vi "Seq Edit Step.vi"(6 "config paths":T1, 8 "Error In":errorcluster, 9 "Segment Info In":T2, 10 "Basic Steps":string[](array[string]), 11 "VI Names":string[](array[string])) -> (0 "Error Out":errorcluster, 1 "Step Hisitory":string[](array[string]), 2 "Segment Info Out":T2, 3 "Add Step?":bool)   [LabVIEW 2018]
uses:
  type defs/Sequence Info.ctl
  type defs/config paths for seq def.ctl
panel:
  out "File Name":string
  out "file or folder exists?":bool
  out "appended path":path
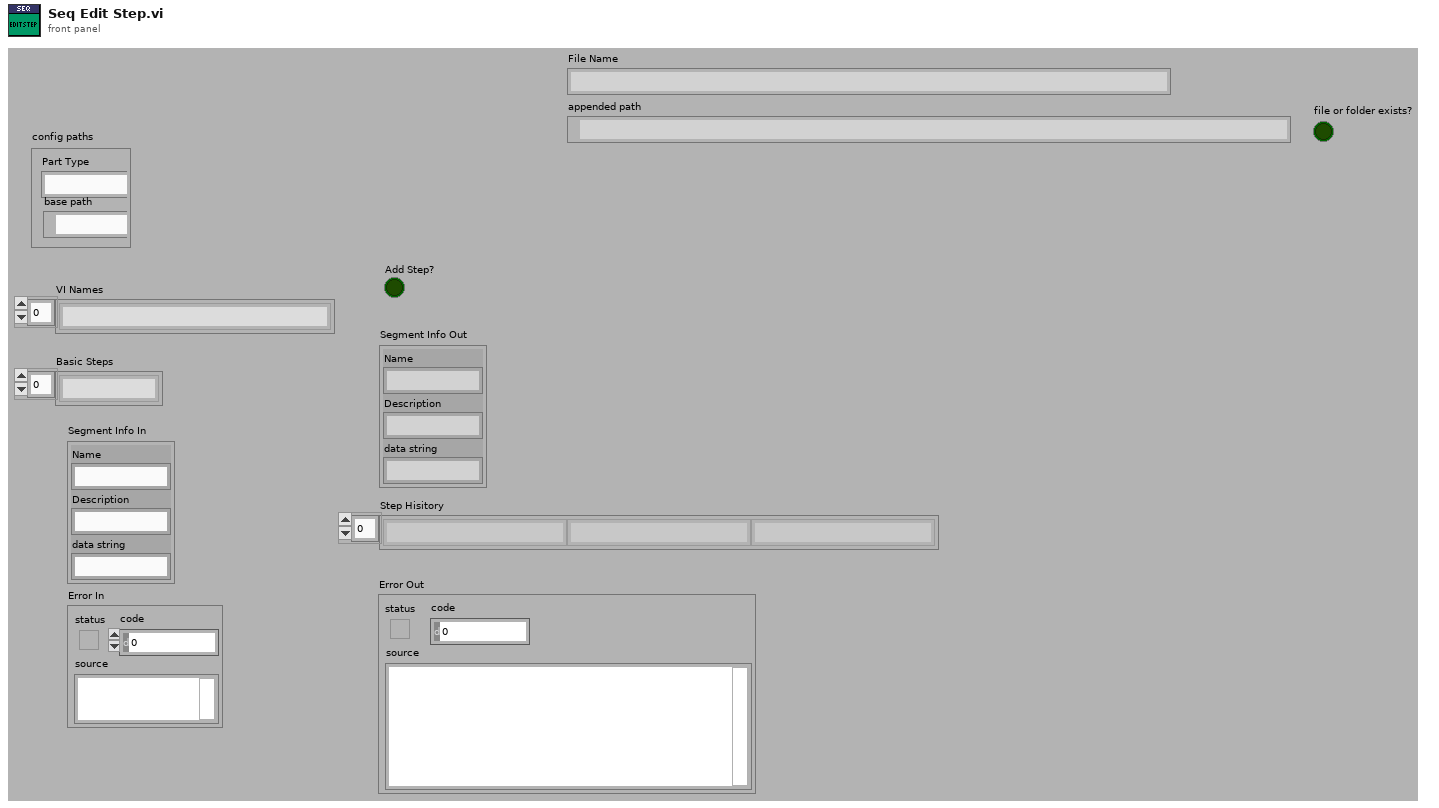
[diagram p1: front panel]
types:
  T1 = typedef "config paths for seq def.ctl" = cluster{"Part Type":string, "base path":path}
  T2 = typedef "Sequence Info.ctl" = cluster{"Name":string, "Description":string, "data string":string}
  T3 = enum32{"Invalid", "Standard", "Closed", "Hidden", "Minimized", "Maximized"}
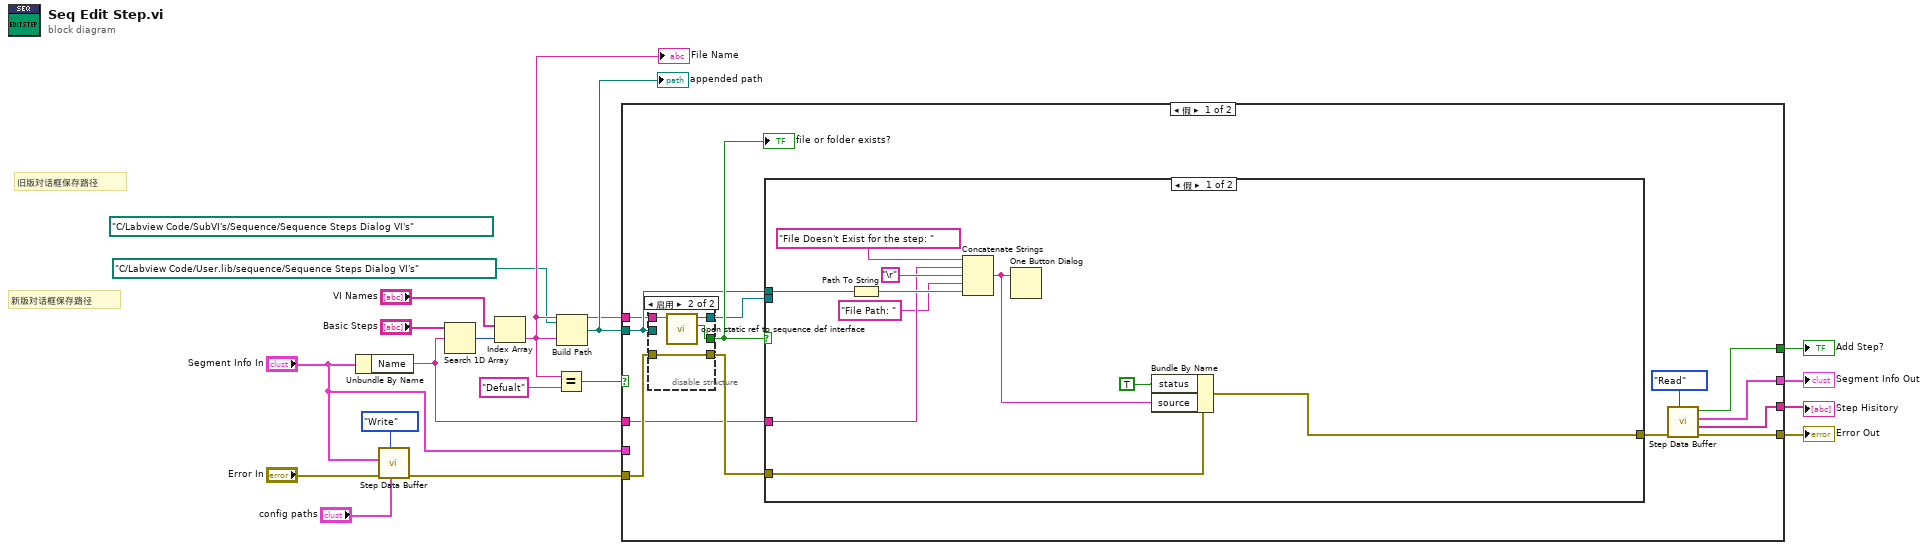
[diagram p0: block diagram]
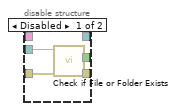
[diagram p2: hidden frame]
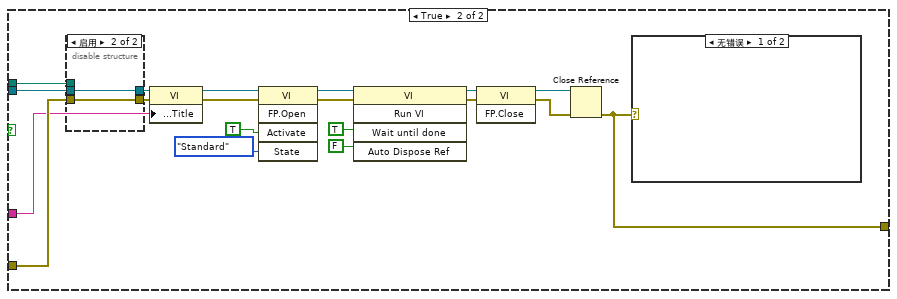
[diagram p3: hidden frame]
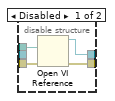
[diagram p4: hidden frame]
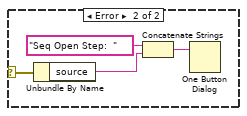
[diagram p5: hidden frame]
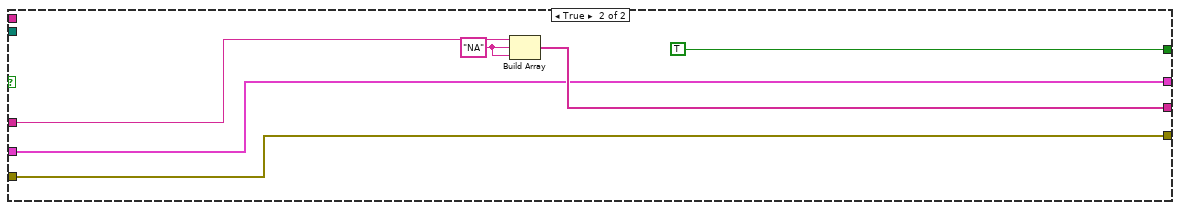
[diagram p6: hidden frame]
diagram:
  (unwired) path "C:/Labview Code/SubVI's/Sequence/Sequence Steps Dialog VI's"
  # "新版对话框保存路径"
  # "旧版对话框保存路径"
  n1 = Unbundle By Name("Segment Info In") -> ("Name"=w14:string)
  n2 = call "Step Data Buffer.vi"("config paths"="config paths", "Mode"=enum16{"Init", "Read", "Write"}."Write", "Error In"="Error In", "Segment Data In"="Segment Info In") -> ("Error Out"=w11:errorcluster)  [unwired: 3 in, 4 out]
  n3 = Search 1D Array(1D array="Basic Steps", element=w14) -> (index of element=w10:i32)  [unwired: 1 in]
  n4 = Index Array(array="VI Names", index=w10) -> (element=w2:string)
  "File Name" <- w2
  n5 = Equal?(x=w2, y="Defualt") -> (x = y?=w8:bool)
  n6 = Build Path(base path=path "C:/Labview Code/User.lib/sequence/Sequence Steps Dialog VI's", name or relative path=w2) -> (appended path=w7:path)
  "appended path" <- w7
  n7 = case shown="假" w8 {
    tunnel: w7 -> [w30 _]
    tunnel: w11 -> [w29 w81]
    tunnel: [w25 w81] -> w15
    tunnel: w14 -> [w21 w83]
    tunnel: [w24 w82] -> w18
    tunnel: [w22 TRUE ("Add Step?")] -> w6
    tunnel: "Segment Info In" -> [_ w79]
    tunnel: [w23 w79] -> w4
    tunnel: w2 -> [w20 _]
    frame False {
      n8 = disable-structure shown="启用" {
        disable-tunnel: [w35 w37] -> w31
        disable-tunnel: w30 -> [w34 _]
        disable-tunnel: w29 -> [w33 w39]
        disable-tunnel: [w32 w39] -> w28
        disable-tunnel: w20 -> [_ w38]
        disable-tunnel: [_ w36] -> w19
        frame Disabled {
          n9 = call <vilib>:"Check if File or Folder Exists.vi"("error in (no error)"=w33, "path"=w34) -> ("error out"=w32:errorcluster, "file or folder exists?"=w35:bool)  [unwired: 7 in, 1 out]
        }
        frame Enabled {
          n10 = call "open static ref to sequence def interface.vi"("vi name"=w38) -> ("exists"=w37:bool, "VI out"=w36:refnum<vi>)  [unwired: 9 in]
        }
      }
      "file or folder exists?" <- w31
      n11 = case shown="假" w31 {
        tunnel: w30 -> [w49 w68]
        tunnel: [w42 w51] -> w26
        tunnel: w28 -> [w43 w67]
        tunnel: w21 -> [w45 w54]
        tunnel: w19 -> [_ w50]
        frame False {
          n12 = Path To String(path=w49) -> (string=w48:string)
          n13 = Concatenate Strings("File Doesn't Exist for the step: " ("string"), w45, "\r", "File Path: " ("string"), w48) -> (w41:string)
          n14 = One Button Dialog(message=w41) -> ()  [unwired: 1 in, 1 out]
          n15 = Bundle By Name(cluster=w43, "status"=TRUE, "source"=w41) -> (w42:errorcluster)
        }
        frame True {
          n16 = disable-structure shown="启用" {
            disable-tunnel: w68 -> [w72 _]
            disable-tunnel: w67 -> [w71 w74]
            disable-tunnel: [w70 w73] -> w58
            disable-tunnel: [w69 w74] -> w57
            disable-tunnel: w50 -> [_ w73]
            frame Disabled {
              n17 = Open VI Reference(vi path=w72, error in (no error)=w71) -> (vi reference=w70:refnum<vi>, error out=w69:errorcluster)  [unwired: 4 in]
            }
            frame Enabled {
            }
          }
          n18 = property class="VI"(reference=w58, error in=w57, "Front Panel.Title"=w54) -> (reference out=w55:refnum<vi>, error out=w56:errorcluster)
          n19 = invoke class="VI" method="FP.Open"(reference=w55, error in=w56, "Activate"=TRUE ("Activate?"), "State"=T3."Standard") -> (reference out=w62:refnum<vi>, error out=w59:errorcluster)  [unwired: 1 in, 3 out]
          n20 = invoke class="VI" method="Run VI"(reference=w62, error in=w59, "Wait until done"=TRUE ("Wait Until Done"), "Auto Dispose Ref"=FALSE ("Auto Dispose Reference")) -> (reference out=w61:refnum<vi>, error out=w60:errorcluster)  [unwired: 1 in, 3 out]
          n21 = invoke class="VI" method="FP.Close"(reference=w61, error in=w60) -> (reference out=w53:refnum<vi>, error out=w52:errorcluster)  [unwired: 1 in, 1 out]
          n22 = Close Reference(reference=w53, error in (no error)=w52) -> (error out=w51:errorcluster)
          n23 = case shown="无错误" w51 {
            selector: w51 -> [_ w77]
            frame No Error {
            }
            frame Error {
              n24 = Unbundle By Name(w77) -> ("source"=w75:string)
              n25 = Concatenate Strings("Seq Open Step:  " ("message"), w75) -> (w76:string)
              n26 = One Button Dialog(message=w76) -> ()  [unwired: 1 in, 1 out]
            }
          }
        }
      }
      n27 = call "Step Data Buffer.vi"("Mode"=enum16{"Init", "Read", "Write"}."Read", "Error In"=w26) -> ("Error Out"=w25:errorcluster, "Step Hisitory Out"=w24:string[], "Segment Data Out"=w23:T2, "Add Step? Out"=w22:bool)  [unwired: 5 in, 1 out]
    }
    frame True {
      w84 = "NA" ("element")
      n28 = Build Array(w83, w84, w84) -> (w82:string[])
    }
  }
  "Step Hisitory" <- w18
  "Segment Info Out" <- w4
  "Add Step?" <- w6
  "Error Out" <- w15
